vi "status.vi"(8 "errorIn":errorcluster, 11 "refer":refnum<queue>) -> (0 "errorOut":errorcluster, 2 "numWaitToProcess":i32, 3 "refer":refnum<queue>)   [LabVIEW 2017]
doc: "refer：队列索引\nnumWaitToProcess：等待处理的消息数量"
uses:
  models/EMSGData.ctl
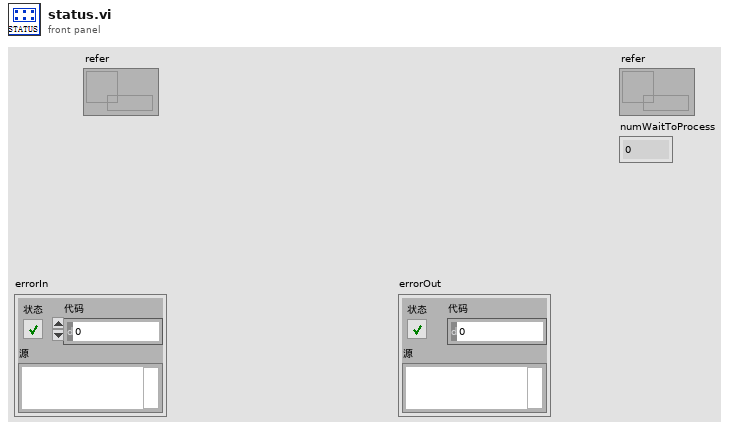
[diagram p1: front panel]
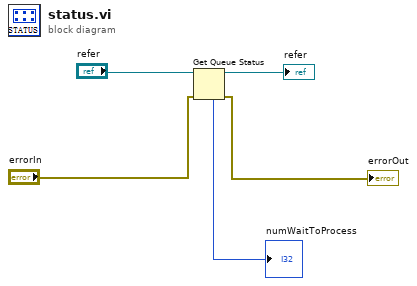
[diagram p0: block diagram]
diagram:
  n1 = Get Queue Status(queue="refer", error in (no error)="errorIn") -> (queue out=→"refer":refnum<queue>, error out=→"errorOut":errorcluster, # elements in queue=→"numWaitToProcess":i32)  [unwired: 1 in, 5 out]
